vi "Execute Test Suite.vi"(8 "error in (no error)":errorcluster, 10 "Test Suite":refnum<class "LUnit Test Suite.lvclass">, 11 "Execution API in":refnum<class "Execution API.lvclass">) -> (0 "error out":errorcluster, 3 "Execution API out":refnum<class "Execution API.lvclass">)   [LabVIEW 2020, in "Execution API.lvclass"]
uses:
  Execution API.lvclass
  Test Suite/LUnit Test Suite.lvclass
  Execution API.lvclass/Execution API.ctl
  Application Framework/Process Classes/Process/Process.lvclass/Process.ctl
  Application Framework/Process Classes/Process/Protected/Messaging/Enqueue Message.vi
  Test Runner/Test Runner.lvclass
  C:/Users/anton/Documents/GitHub/LUnit/source/Application Framework/Process Classes/Process/Process.lvclass
  Report Generator/Report Generator.lvclass
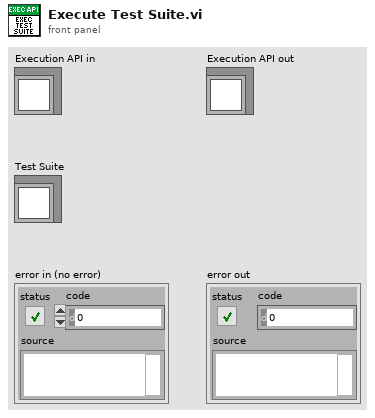
[diagram p1: front panel]
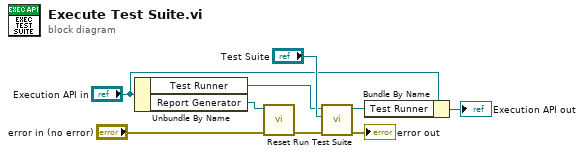
[diagram p0: block diagram]
diagram:
  n1 = Unbundle By Name("Execution API in") -> ("Test Runner"=w2:refnum<class "Test Runner.lvclass">, "Report Generator"=w9:refnum<class "Report Generator.lvclass">)
  n2 = call "Reset.vi"("error in (no error)"="error in (no error)", "Report Generator In"=w9) -> ("error out"=w3:errorcluster)  [unwired: 8 in, 1 out]
  n3 = call "Run Test Suite.vi"("error in (no error)"=w3, "Test Suite In"="Test Suite", "Test Runner In"=w2) -> ("error out"=→"error out":errorcluster, "Test Runner Out"=w1:refnum<class "Test Runner.lvclass">)  [unwired: 7 in]
  n4 = Bundle By Name(cluster="Execution API in", "Test Runner"=w1) -> (→"Execution API out":refnum<class "Execution API.lvclass">)
